vi "fgv_GSlam_matrix-buffer.vi"(7 "cmd":enum16{"write H", "write inv(H)", "read"}(ring), 10 "H inv":T1, 11 "H":T1) -> (2 "H inv out":T1 caption="H inv", 3 "H out":T1)   [LabVIEW 2019]
uses:
  <vilib>/Analysis/Matrix/Datatypes/RealMatrix.ctl
  <vilib>/Analysis/Matrix/NI_Matrix.lvlib
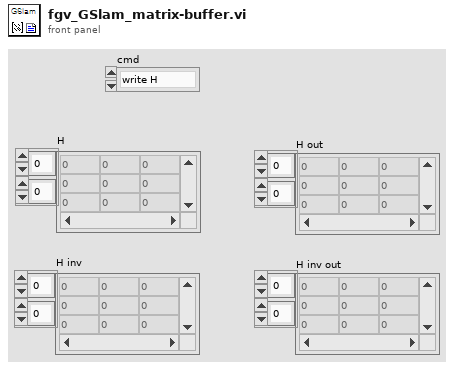
[diagram p1: front panel]
types:
  T1 = typedef "NI_Matrix.lvlib/RealMatrix.ctl" = dbl[][]
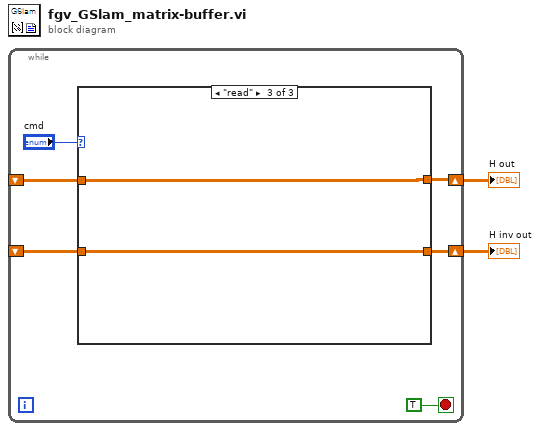
[diagram p0: block diagram]
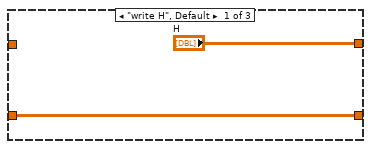
[diagram p2: hidden frame]
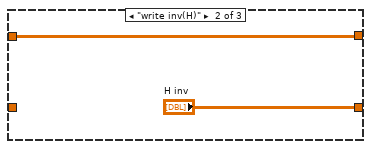
[diagram p3: hidden frame]
diagram:
  n1 = while {
    shift-right: [w5] -> w2
    shift-left: _ -> [w3]
    shift-right: [w6] -> w1
    shift-left: _ -> [w4]
    stop <- TRUE stop-if-true
    n2 = case shown="\"read\"" "cmd" {
      tunnel: [w9 "H inv" w14] -> w6
      tunnel: ["H" w11 w13] -> w5
      tunnel: w4 -> [w9 _ w14]
      tunnel: w3 -> [_ w11 w13]
      frame "write H", Default {
      }
      frame "write inv(H)" {
      }
      frame "read" {
      }
    }
  }
  "H out" <- w2
  "H inv out" <- w1
